vi "JS Chart.vi"() -> ()   [LabVIEW 2024]
uses:
  <vilib>/sklein/WebView2/Webview2 Control/WebView2 Control.xctl
panel:
  out "Timed Out":bool
  in  "Chart Label":string
  in  "Stop":bool
  out "Chart":string(xcontrol)
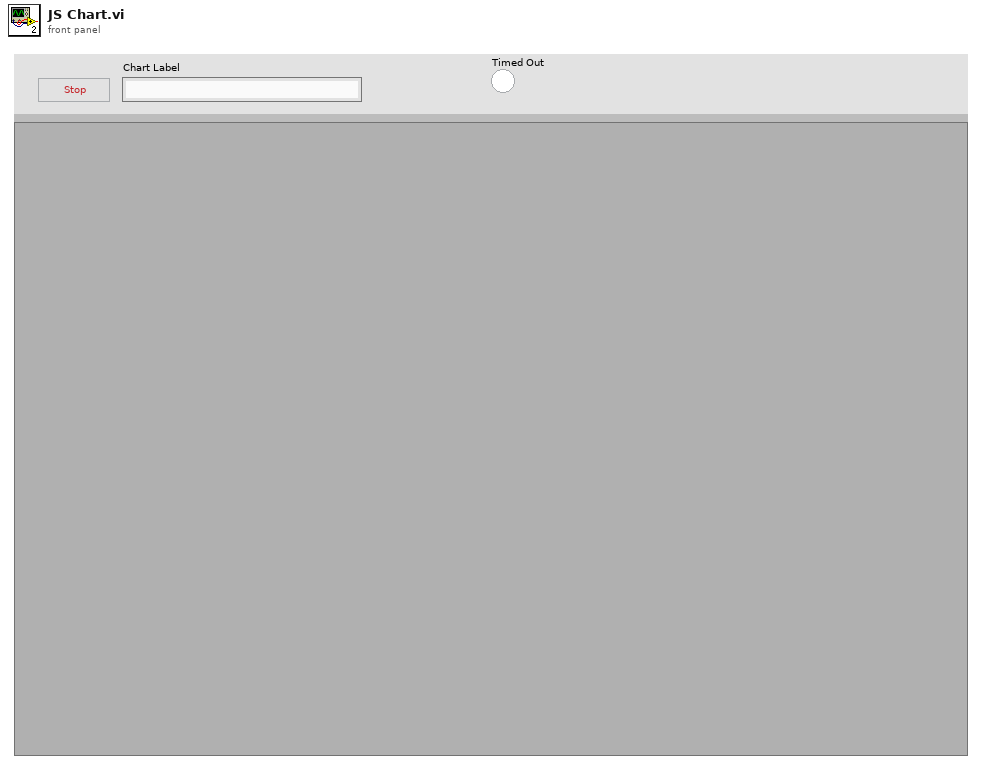
[diagram p1: front panel]
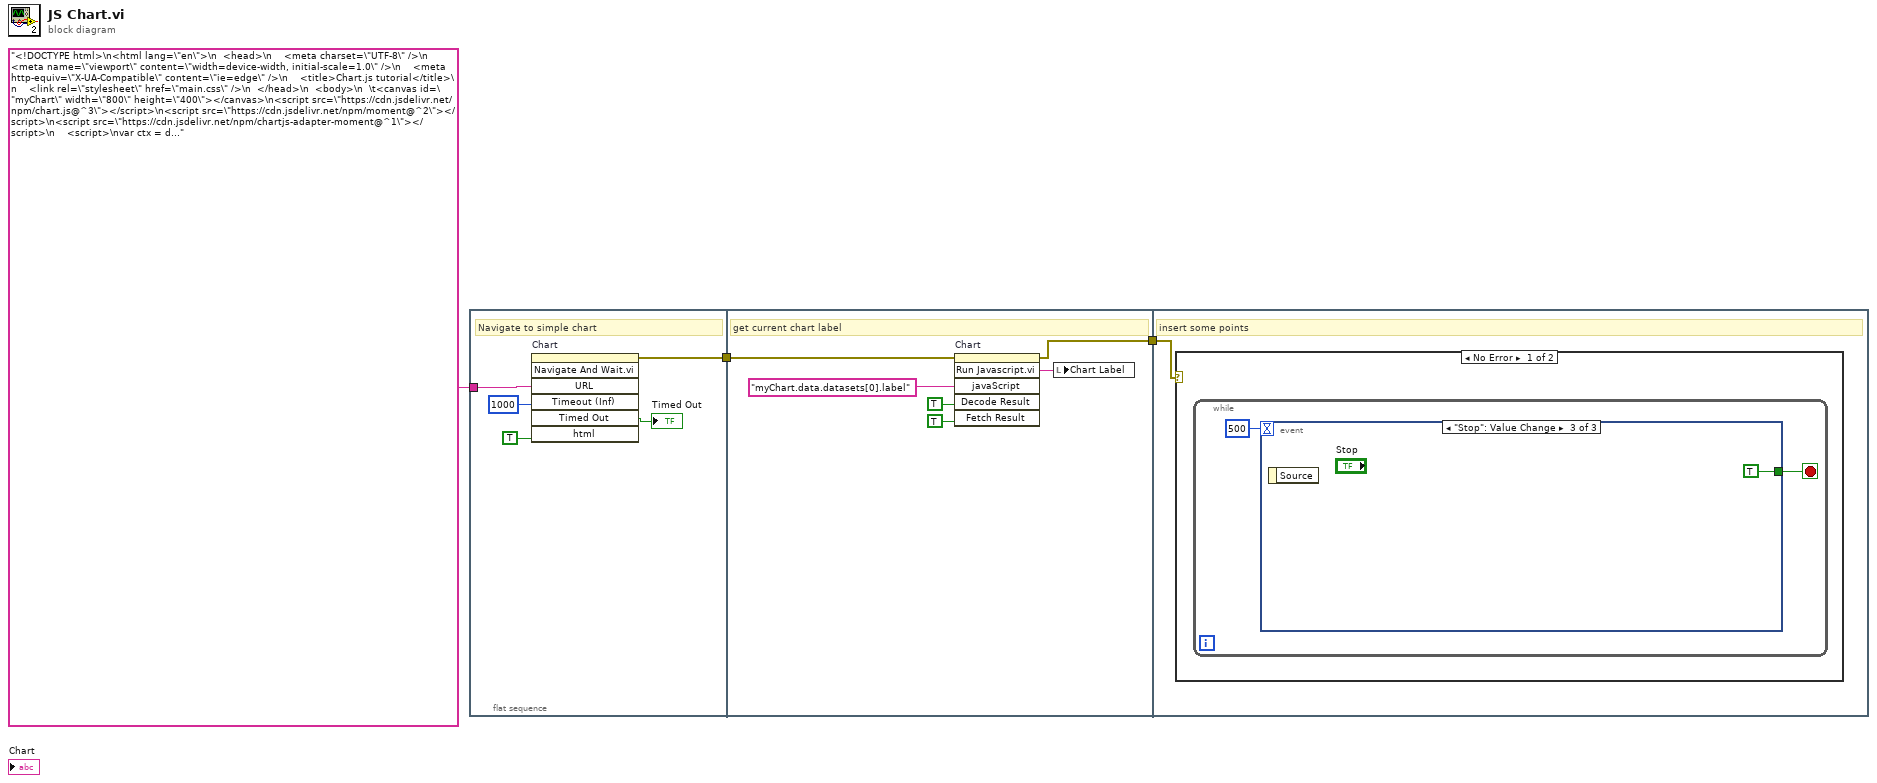
[diagram p0: block diagram]
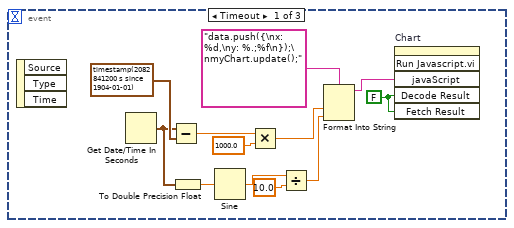
[diagram p2: hidden frame]
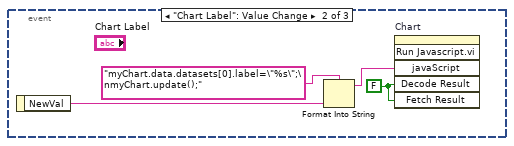
[diagram p3: hidden frame]
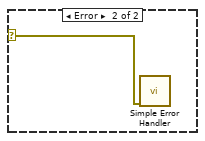
[diagram p4: hidden frame]
diagram:
  n1 = flat-sequence {
    tunnel: "<!DOCTYPE html>\n<html lang=\"en\">\n  <head>\n    <meta charset=\"UTF-8\" />\n    <meta name=\"viewport\" content=\"width=device-width, initial-scale=1.0\" />\n    <meta http-equiv=\"X-UA-Compatible\" content=\"ie=edge\" />\n    <title>Chart.js tutorial</title>\n    <link rel=\"stylesheet\" href=\"main.css\" />\n  </head>\n  <body>\n  \t<canvas id=\"myChart\" width=\"800\" height=\"400\"></canvas>\n<script src=\"https://cdn.jsdelivr.net/npm/chart.js@^3\"></script>\n<script src=\"https://cdn.jsdelivr.net/npm/moment@^2\"></script>\n<script src=\"https://cdn.jsdelivr.net/npm/chartjs-adapter-moment@^1\"></script>\n    <script>\nvar ctx = document.getElementById(\"myChart\");\n\nvar data = []\n\nvar myChart = new Chart(ctx, {\n type: \"line\",\n options: {\n\tscales: {\n\t\tx: {\n\t\t\ttype: 'time'\n\t\t}\n\t}\n },\n data: {\n    datasets: [\n    {\n\t\tlabel: \"Data\",\n        data: data,\n        backgroundColor: \"rgba(255, 99, 132, 0.2)\",\n        borderColor: \"rgba(255, 99, 132, 1)\",\n        borderWidth: 1\n    }\n    ]\n }\n});\n\n\t</script>\n  </body>\n</html>\n" -> [w5]
    tunnel: [w4] -> w1
    tunnel: [w11] -> w3
    tunnel: w1 -> [w9]
    tunnel: w3 -> [w15]
    frame #0 {
      # "Navigate to simple chart"
      n2 = invoke on="Chart" class="WebView2 Control (strict)" method="Navigate And Wait.vi"("URL"=w5, "Timeout (Inf)"=1000, "html"=TRUE) -> (error out=w4:errorcluster, "Timed Out"=→"Timed Out":bool)  [unwired: 4 in, 5 out]
    }
    frame #1 {
      # "get current chart label"
      n3 = invoke on="Chart" class="WebView2 Control (strict)" method="Run Javascript.vi"(error in=w9, "javaScript"="myChart.data.datasets[0].label", "Decode Result"=TRUE, "Fetch Result"=TRUE) -> (error out=w11:errorcluster, "Run Javascript.vi"=w12:string)  [unwired: 2 in, 4 out]
      n4 = local write "Chart Label"(w12) -> ()
    }
    frame #2 {
      # "insert some points"
      n5 = case shown="No Error" w15 {
        selector: w15 -> [_ w35]
        frame No Error {
          n6 = while {
            stop <- w16 stop-if-true
            n7 = event shown="[2] \"Stop\": Value Change" {
              selector: _ -> [_ _ _]
              dyn-events: _ -> [_ _ _]
              timeout: 500 -> [_ _ _]
              tunnel: [_ _ TRUE] -> w16
              event Timeout {
                w18 = FALSE ("Decode Result")
                n8 = event-data() -> ()  [unwired: 1 in, 3 out]
                n9 = Get Date/Time In Seconds() -> (seconds since 1Jan1904=w20:timestamp)
                n10 = Subtract(x=w20, y=timestamp(2082841200 s since 1904-01-01) ("current time")) -> (x-y=w22:dbl)
                n11 = To Double Precision Float(number=w20) -> (double precision float=w27:dbl)
                n12 = Sine(x=w27) -> (sin(x)=w26:dbl)
                n13 = Multiply(x=w22, y=1000.0) -> (x*y=w19:dbl)
                n14 = Divide(x=w26, y=10.0) -> (x/y=w25:dbl)
                n15 = Format Into String(format string="data.push({\nx: %d,\ny: %.;%f\n});\nmyChart.update();" ("javaScript"), w19, w25) -> (resulting string=w28:string)  [unwired: 2 in, 1 out]
                n16 = invoke on="Chart" class="WebView2 Control (strict)" method="Run Javascript.vi"("javaScript"=w28, "Decode Result"=w18, "Fetch Result"=w18) -> ()  [unwired: 3 in, 6 out]
              }
              event "Chart Label": Value Change {
                w30 = FALSE ("Decode Result")
                n17 = event-data() -> ("NewVal"=w31:string)  [unwired: 1 in]
                n18 = Format Into String(format string="myChart.data.datasets[0].label=\"%s\";\nmyChart.update();" ("javaScript"), w31) -> (resulting string=w32:string)  [unwired: 2 in, 1 out]
                n19 = invoke on="Chart" class="WebView2 Control (strict)" method="Run Javascript.vi"("javaScript"=w32, "Decode Result"=w30, "Fetch Result"=w30) -> ()  [unwired: 3 in, 6 out]
              }
              event "Stop": Value Change {
                n20 = event-data() -> ()  [unwired: 1 in, 1 out]
              }
            }
          }
        }
        frame Error {
          n21 = call <vilib>:"Simple Error Handler.vi"("error in (no error)"=w35) -> ()  [unwired: 4 in, 5 out]
        }
      }
    }
  }
